vi "Open Device.vi"(8 "error in":errorcluster, 10 "Serial Number":string) -> (0 "error out":errorcluster, 3 "reference out":refnum<k24>)   [LabVIEW 2020, in "Topas4.lvlib"]
uses:
  Topas4.lvlib
  C:/Windows/SysWOW64/Topas4Lib.dll
  Windows/SysWOW64/Topas4Lib.dll
  <vilib>/Utility/error.llb/Error Cluster From Error Code.vi
  <vilib>/ErrorRing/Error Ring.xnode
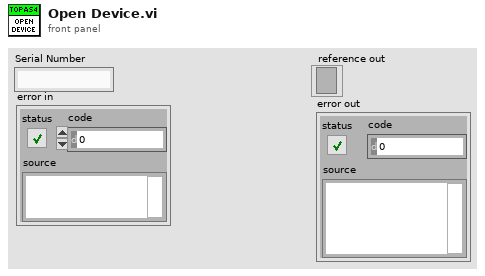
[diagram p1: front panel]
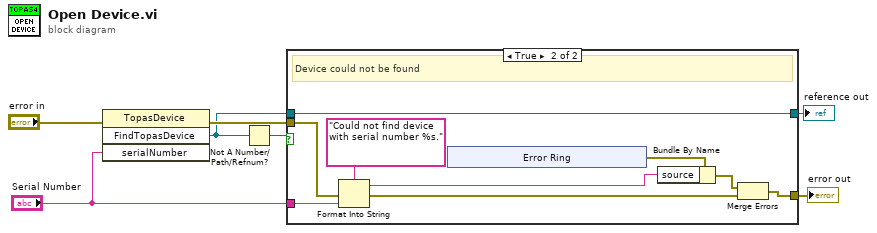
[diagram p0: block diagram]
diagram:
  n1 = invoke class="TopasDevice" method="FindTopasDevice"(error in="error in", "serialNumber"="Serial Number") -> (error out=w5:errorcluster, "FindTopasDevice"=w1:refnum<k24>)  [unwired: 2 in, 2 out]
  n2 = Not A Number/Path/Refnum?(number/path/refnum=w1) -> (NaN/Path/Refnum?=w7:bool)
  n3 = case shown="True" w7 {
    tunnel: "Serial Number" -> [_ w18]
    tunnel: w5 -> [w8 w17]
    tunnel: [w8 w12] -> w2
    tunnel: w1 -> [w9 w10]
    tunnel: [w9 w10] -> w3
    frame False {
      # "no error. device found"
    }
    frame True {
      # "Device could not be found"
      n4 = Format Into String(format string="Could not find device with serial number %s.", error in=w17, w18) -> (resulting string=w13:string, error out=w16:errorcluster)  [unwired: 1 in]
      n5 = xnode "Error Ring"() -> ("error out"=w14:errorcluster)
      n6 = Bundle By Name(cluster=w14, "source"=w13) -> (w11:errorcluster)
      n7 = Merge Errors(w11, w16) -> (w12:errorcluster)
    }
  }
  "reference out" <- w3
  "error out" <- w2
